vi "Scale Columns (Ratio).vi"(8 "error in (no error)":errorcluster, 10 "Column Widths [unitless ratio]":dbl[](array[numeric]), 11 "MulticolumnListbox in":refnum<vi>) -> (0 "error out":errorcluster)   [LabVIEW 2018, in "MVA Framework.lvlib" / "ListboxExtensions.lvlib"]
doc: "缩放列（比率）"
uses:
  ListboxExtensions.lvlib
  <vilib>/Utility/miscctls.llb/LVRowAndColumnTypeDef.ctl
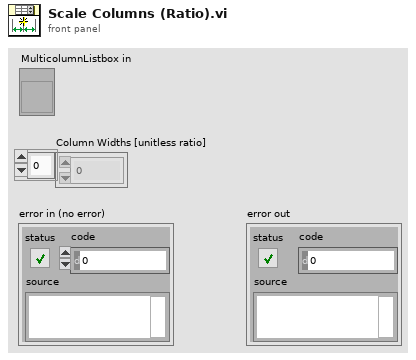
[diagram p1: front panel]
types:
  T1 = typedef "LVRowAndColumnTypeDef.ctl" = cluster{"Row":i32, "Column":i32}
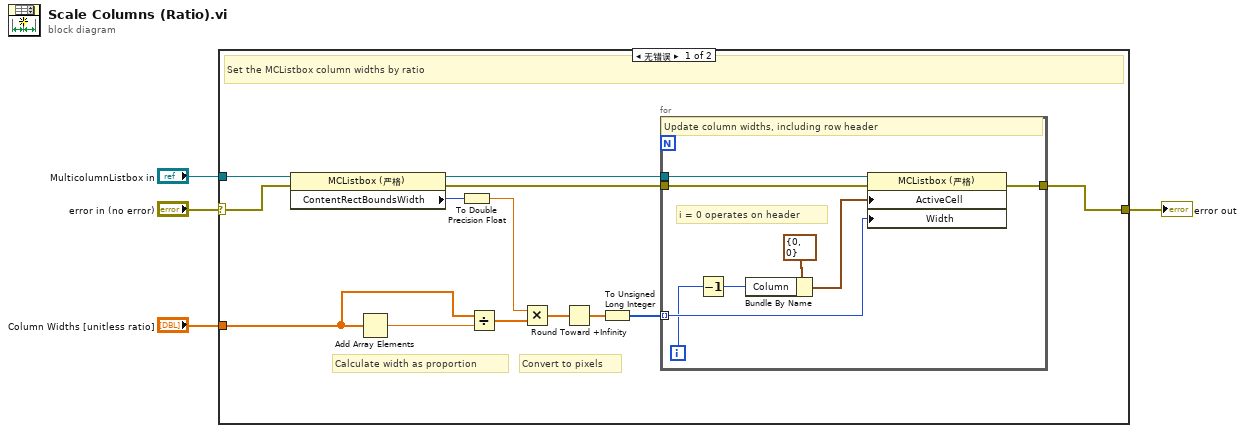
[diagram p0: block diagram]
diagram:
  n1 = case shown="无错误" "error in (no error)" {
    selector: "error in (no error)" -> [w7 w26]
    tunnel: "Column Widths [unitless ratio]" -> [w5 _]
    tunnel: "MulticolumnListbox in" -> [w9 _]
    tunnel: [w6 w26] -> w4
    frame No Error {
      # "Convert to pixels"
      # "Calculate width as proportion"
      # "Set the MCListbox column widths by ratio"
      n2 = property class="MCListbox (严格)"(reference=w9, error in=w7) -> (reference out=w16:refnum<vi>, error out=w8:errorcluster, "ContentRectBoundsWidth"=w15:i32)
      n3 = Add Array Elements(numeric array=w5) -> (sum=w17:dbl)
      n4 = To Double Precision Float(number=w15) -> (double precision float=w10:dbl)
      n5 = Divide(x=w5, y=w17) -> (x/y=w14:dbl[])
      n6 = Multiply(x=w10, y=w14) -> (x*y=w13:dbl[])
      n7 = Round Toward +Infinity(x=w13) -> (ceil(x): smallest int >= x=w12:dbl[])
      n8 = To Unsigned Long Integer(number=w12) -> (unsigned 32bit integer=w11:u32[])
      n9 = for {
        tunnel: [w25] -> w6
        tunnel: w16 -> [w24]
        tunnel: w11 -> [w21] mode=indexing
        tunnel: w8 -> [w19]
        i -> [w18]
        # "i = 0 operates on header"
        # "Update column widths, including row header"
        n10 = Decrement(x=w18) -> (x-1=w20:i32)
        n11 = Bundle By Name(cluster=T1 {"Row"=0, "Column"=0} ("Active Cell:Active Cell"), "Column"=w20) -> (w22:T1)
        n12 = property class="MCListbox (严格)"(reference=w24, error in=w19, "ActiveCell"=w22, "Width"=w21) -> (error out=w25:errorcluster)  [unwired: 1 out]
      }
    }
    frame Error {
      # "Do nothing to the MCListbox if error in"
    }
  }
  "error out" <- w4
